vi "Connect Case Selector Terminal.vi"(8 "error in (no error)":errorcluster, 10 "Wire Source":refnum<vi>, 11 "Case Structure in":refnum<vi>) -> (0 "error IO":errorcluster, 3 "Case Structure out":refnum<vi>)   [LabVIEW 2019, in "VI Scripting Utilities.lvlib"]
uses:
  VI Scripting Utilities.lvlib
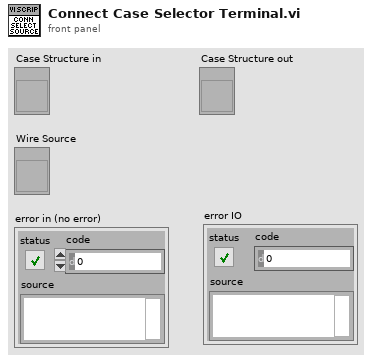
[diagram p1: front panel]
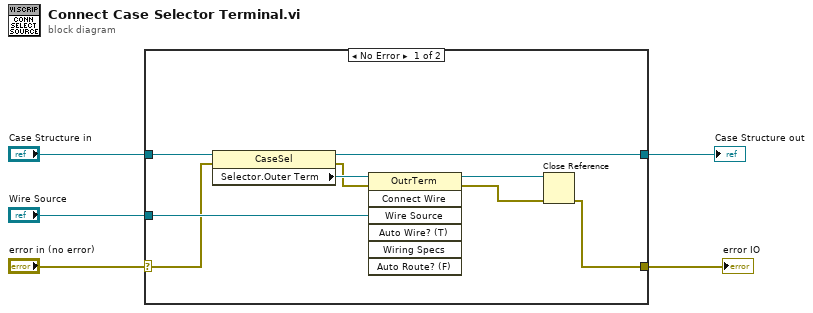
[diagram p0: block diagram]
diagram:
  n1 = case shown="No Error" "error in (no error)" {
    selector: "error in (no error)" -> [w9 w16]
    tunnel: "Wire Source" -> [w14 _]
    tunnel: "Case Structure in" -> [w11 w15]
    tunnel: [w10 w15] -> w2
    tunnel: [w6 w16] -> w1
    frame No Error {
      n2 = property class="CaseSel"(reference=w11, error in=w9) -> (reference out=w10:refnum<vi>, error out=w7:errorcluster, "Selector.Outer Term"=w8:refnum<vi>)
      n3 = invoke class="OutrTerm" method="Connect Wire"(reference=w8, error in=w7, "Wire Source"=w14) -> (reference out=w12:refnum<vi>, error out=w13:errorcluster)  [unwired: 4 in, 5 out]
      n4 = Close Reference(reference=w12, error in (no error)=w13) -> (error out=w6:errorcluster)
    }
    frame Error {
    }
  }
  "Case Structure out" <- w2
  "error IO" <- w1
